vi "emi_Tile Gradient Image.vi"(0 "image data Inn":T1, 5 "Width(400)":i32=400, 9 "Height(600)":i32=600, 11 "error in (no error)":errorcluster) -> (4 "image data Tiled":T1, 8 "Picture":picture, 15 "error out":errorcluster)   [LabVIEW 2011]
doc: "Input an image and a width and hight.\n\nAn image will be created where the original image is tiled veritcaky until with is reached,\nThe bottum most line will be repesaded horizontaly,until height is reached.\n\nOn Error:No action"
uses:
  <vilib>/picture/picture.llb/imagedata.ctl
panel:
  out "Stop color":u32
  out "Start color":u32
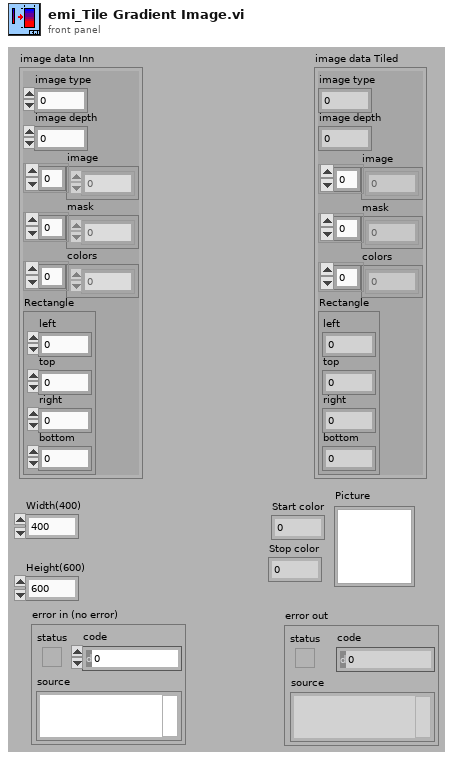
[diagram p1: front panel]
types:
  T1 = typedef "imagedata.ctl" = cluster{"image type":i32, "image depth":i32, "image":u8[], "mask":u8[], "colors":u32[], "Rectangle":cluster{"left":i16, "top":i16, "right":i16, "bottom":i16}}
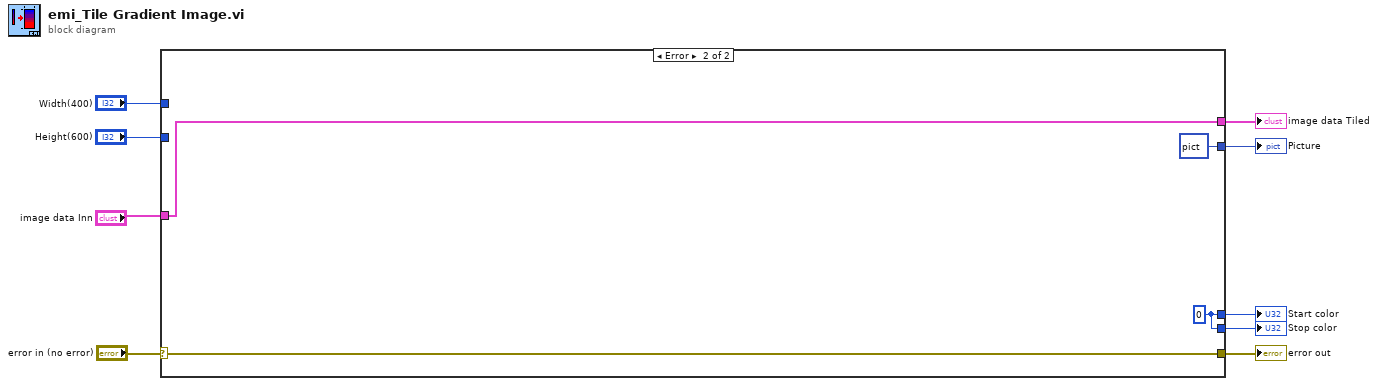
[diagram p0: block diagram]
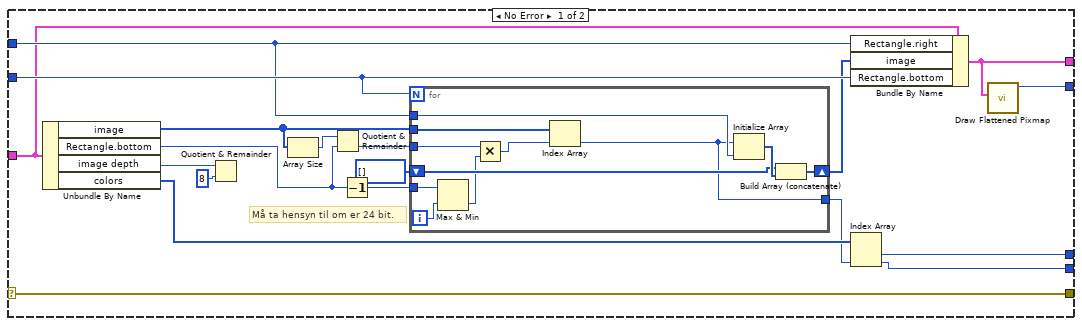
[diagram p2: hidden frame]
diagram:
  n1 = case shown="Error" "error in (no error)" {
    selector: "error in (no error)" -> [w10 w42]
    tunnel: "Height(600)" -> [w21 _]
    tunnel: "Width(400)" -> [w20 _]
    tunnel: [w16 w40] -> w7
    tunnel: [w15 w40] -> w6
    tunnel: [w13 w43] -> w5
    tunnel: [w12 picture data[5B] ("new picture")] -> w4
    tunnel: "image data Inn" -> [w11 w43]
    tunnel: [w10 w42] -> w1
    frame No Error {
      # "Må ta hensyn til om er 24 bit."
      n2 = Unbundle By Name(w11) -> ("image"=w22:u8[], "Rectangle.bottom"=w25:i16, "image depth"=w27:i32, "colors"=w17:u32[])
      n3 = Quotient & Remainder(x=w27, y=8) -> ()  [unwired: 2 out]
      n4 = Array Size(array=w22) -> (size(s)=w24:i32)
      n5 = Quotient & Remainder(x=w24, y=w25) -> (floor(x/y)=w23:i32)  [unwired: 1 out]
      n6 = Decrement(x=w25) -> (x-1=w26:i16)
      n7 = for {
        N: w21 -> [_]
        tunnel: w22 -> [w37]
        shift-right: [w38] -> w19
        shift-left: u8[] [] -> [w36]
        tunnel: w20 -> [w30]
        tunnel: w23 -> [w34]
        tunnel: w26 -> [w35]
        tunnel: [w29] -> w14
        i -> [w33]
        n8 = Max & Min(x=w35, y=w33) -> (min(x,y)=w32:i32)  [unwired: 1 out]
        n9 = Multiply(x=w34, y=w32) -> (x*y=w31:i32)
        n10 = Index Array(array=w37, index=w31) -> (element=w29:u8)
        n11 = Initialize Array(w29, w30) -> (w39:u8[])
        n12 = Build Array (concatenate)(w36, w39) -> (w38:u8[])
      }
      n13 = Bundle By Name(cluster=w11, "Rectangle.right"=w20, "image"=w19, "Rectangle.bottom"=w21) -> (w13:T1)
      n14 = Index Array(array=w17, index #2=w14) -> (element #1=w16:u32, element #2=w15:u32)  [unwired: 1 in]
      n15 = call <vilib>:"Draw Flattened Pixmap.vi"("image data"=w13) -> ("new picture"=w12:picture)  [unwired: 8 in]
    }
    frame Error {
      w40 = u32 0
    }
  }
  "image data Tiled" <- w5
  "Start color" <- w7
  "Stop color" <- w6
  "Picture" <- w4
  "error out" <- w1
